vi "进度条.vi"(9 "文本信息":string, 10 "VISA资源名称":refnum<visa-resource-name>, 11 "Slide输入":refnum<vi>) -> (3 "VISA引用句柄输出":refnum<visa-resource-name>)   [LabVIEW 2016]
panel:
  out "error out":errorcluster
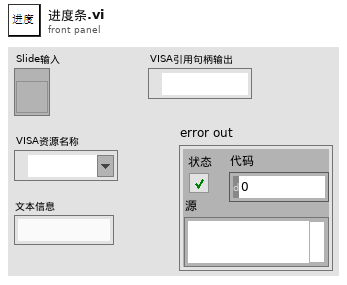
[diagram p1: front panel]
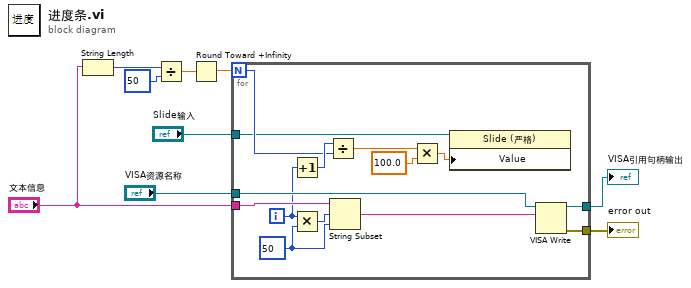
[diagram p0: block diagram]
diagram:
  n1 = String Length(string="文本信息") -> (length=w4:i32)
  n2 = Divide(x=w4, y=50) -> (x/y=w8:dbl)
  n3 = Round Toward +Infinity(x=w8) -> (ceil(x): smallest int >= x=w9:dbl)
  n4 = for {
    N: w9 -> [w17]
    tunnel: "VISA资源名称" -> [w23]
    tunnel: [w22] -> w3
    tunnel: "文本信息" -> [w21]
    tunnel: "Slide输入" -> [w11]
    tunnel: [w10] -> w1
    i -> [w15]
    w14 = 50 ("y")
    n5 = Increment(x=w15) -> (x+1=w18:i32)
    n6 = Multiply(x=w15, y=w14) -> (x*y=w13:i32)
    n7 = Divide(x=w18, y=w17) -> (x/y=w16:dbl)
    n8 = String Subset(string=w21, offset (0)=w13, length (rest)=w14) -> (substring=w20:string)
    n9 = Multiply(x=w16, y=100.0) -> (x*y=w12:dbl)
    n10 = property class="Slide (严格)"(reference=w11, "Value"=w12) -> ()  [unwired: 1 in, 2 out]
    n11 = VISA Write(VISA resource name=w23, write buffer=w20) -> (VISA resource name out=w22:refnum<visa-resource-name>, error out=w10:errorcluster)  [unwired: 1 in, 1 out]
  }
  "VISA引用句柄输出" <- w3
  "error out" <- w1
